vi "文件IO作业.vi"() -> ()   [LabVIEW 2014]
panel:
  in  "停止":bool
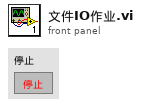
[diagram p1: front panel]
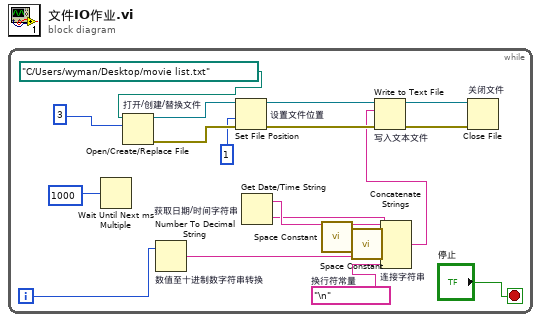
[diagram p0: block diagram]
diagram:
  n1 = while {
    i -> [w13]
    stop <- "停止" stop-if-true
    w10 = "\n"  # 换行符常量
    n2 = Wait Until Next ms Multiple(millisecond multiple=1000) -> ()  [unwired: 1 out]
    n3 = Open/Create/Replace File "打开/创建/替换文件"(file path (use dialog)=path "C:/Users/wyman/Desktop/movie list.txt" ("路径"), operation (0:open)=3) -> (refnum out=w16:refnum<file>, error out=w18:errorcluster)  [unwired: 4 in, 1 out]
    n4 = Number To Decimal String "数值至十进制数字符串转换"(number=w13) -> (decimal integer string=w9:string)  [unwired: 1 in]
    n5 = Set File Position "设置文件位置"(refnum=w16, from (0:start)=1, error in=w18) -> (refnum out=w15:refnum<file>, error out=w19:errorcluster)  [unwired: 1 in]
    n6 = Get Date/Time String "获取日期/时间字符串"() -> (date string=w7:string, time string=w6:string)  [unwired: 3 in]
    n7 = call <vilib>:"Space Constant.vi"() -> ("String"=w1:string)
    n8 = call <vilib>:"Space Constant.vi"() -> ("String"=w8:string)
    n9 = Concatenate Strings "连接字符串"(w7, w1, w6, w8, w9, w10) -> (w5:string)
    n10 = Write to Text File "写入文本文件"(file (use dialog)=w15, text=w5, error in=w19) -> (refnum out=w14:refnum<file>, error out=w17:errorcluster)  [unwired: 1 in, 1 out]
    n11 = Close File "关闭文件"(refnum=w14, error in=w17) -> ()  [unwired: 2 out]
  }
